vi "Get MD5.vi"(8 "error in (no error)":errorcluster, 11 "Item Ref in":T1 format="%.0x") -> (0 "error out":errorcluster, 2 "MD5":string, 3 "Item Ref out":T1 format="%.0x")   [LabVIEW 2017, in "DSF Shared.lvlib"]
uses:
  DSF Shared.lvlib
  <vilib>/NI Veristand/Custom Device API/Custom Device Item Ref.ctl
  <vilib>/NI Veristand/Custom Device API/Get Item Property (String).vi
  <vilib>/NI Veristand/Custom Device API/Custom Device API.lvlib
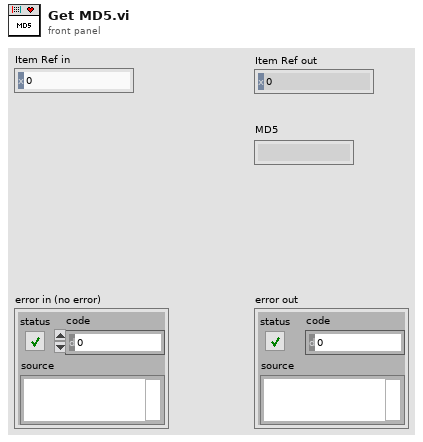
[diagram p1: front panel]
types:
  T1 = typedef "Custom Device API.lvlib/Custom Device Item Ref.ctl" = u64
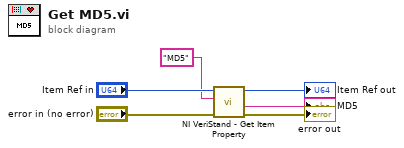
[diagram p0: block diagram]
diagram:
  n1 = call-poly <vilib>:"NI VeriStand - Get Item Property.vi"("error in (no error)"="error in (no error)", "Property Name"="MD5", "Item Ref in"="Item Ref in") -> ("error out"=→"error out":errorcluster, "Value"=→"MD5":string, "Item Ref out"=→"Item Ref out":T1)  [unwired: 5 in, 1 out]
